vi "Read Message Queue.vi"(8 "error in (no error)":errorcluster, 11 "Simple Tree Queue Messenger in":refnum<class "Simple Tree Queue Messenger.lvclass">) -> (0 "error out":errorcluster, 2 "Message Queue":T1, 3 "Simple Tree Queue Messenger out":refnum<class "Simple Tree Queue Messenger.lvclass">)   [LabVIEW 2019, in "Simple Tree Queue Messenger.lvclass"]
uses:
  Simple Tree Queue Messenger.lvclass
  Type Def/Message Queue.ctl
  Ancestor Class/Message/Message.lvclass
  Simple Tree Queue Messenger.lvclass/Simple Tree Queue Messenger.ctl
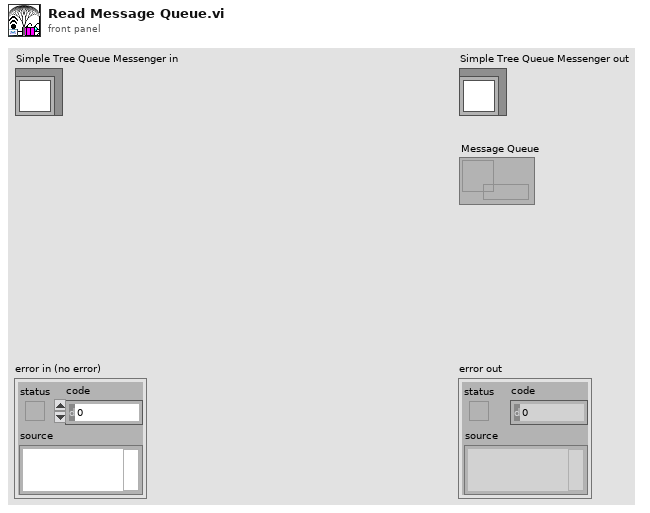
[diagram p1: front panel]
types:
  T1 = typedef "Message Queue.ctl" = refnum<queue>
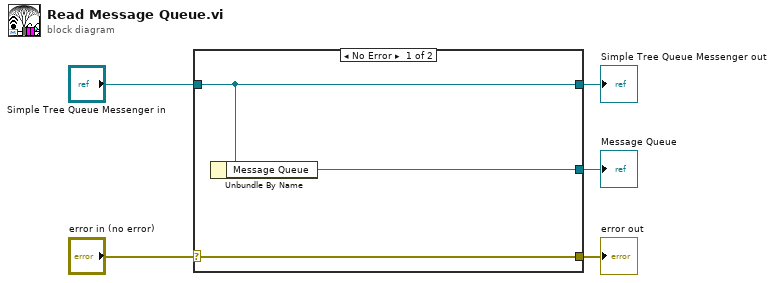
[diagram p0: block diagram]
diagram:
  n1 = case shown="No Error" "error in (no error)" {
    selector: "error in (no error)" -> [w8 w9]
    tunnel: [w8 w9] -> w4
    tunnel: [w7 w10] -> w2
    tunnel: "Simple Tree Queue Messenger in" -> [w7 w10]
    tunnel: [w6 _] -> w1
    frame No Error {
      n2 = Unbundle By Name(w7) -> ("Message Queue"=w6:T1)
    }
    frame Error {
    }
  }
  "error out" <- w4
  "Simple Tree Queue Messenger out" <- w2
  "Message Queue" <- w1
